vi "get_timestamp_from_distance_old.vi"(6 "distance":dbl, 9 "manual end":timestamp, 10 "start":timestamp, 11 "lat/lon position":T1) -> (1 "distance":dbl, 2 "mean speed":dbl, 3 "end times":timestamp[](array[timestamp]), 4 "time between timestamps":dbl)   [LabVIEW 2020]
uses:
  <vilib>/Analysis/1siggen.llb/Ramp Pattern by Delta.vi
  <vilib>/Analysis/NI_AALBase.lvlib
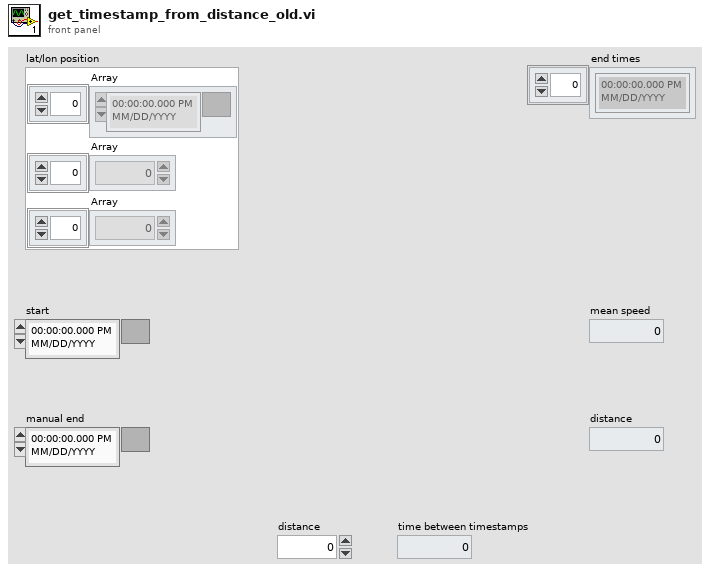
[diagram p1: front panel]
types:
  T1 = cluster{"Array":timestamp[], "Array":dbl[], "Array":dbl[]}
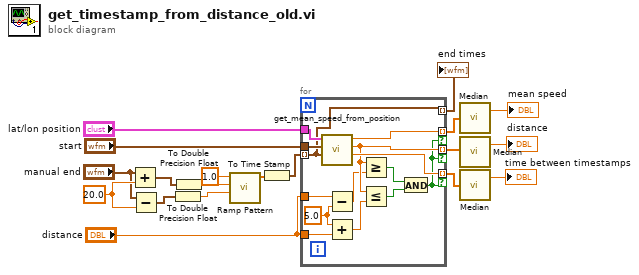
[diagram p0: block diagram]
diagram:
  w5 = 20.0 ("delta")
  n1 = Add(x="manual end", y=w5) -> (x+y=w7:timestamp)
  n2 = Subtract(x="manual end", y=w5) -> (x-y=w8:timestamp)
  n3 = To Double Precision Float(number=w8) -> (double precision float=w9:dbl)
  n4 = To Double Precision Float(number=w7) -> (double precision float=w6:dbl)
  n5 = call-poly <vilib>:"Ramp Pattern.vi"("start"=w9, "end"=w6, "delta"=1.0) -> ("Ramp Pattern"=w10:dbl[])  [unwired: 6 in, 2 out]
  n6 = To Time Stamp(1:w10) -> (0:w11:timestamp[])
  n7 = for {
    tunnel: "start" -> [w33]
    tunnel: "lat/lon position" -> [w32]
    tunnel: w11 -> [w26] mode=indexing
    tunnel: [w31] -> w13 mode=indexing if=w25
    tunnel: [w28] -> w14 mode=indexing if=w25
    tunnel: [w30] -> w15 mode=indexing if=w25
    tunnel: [w26] -> w12 mode=indexing
    tunnel: "distance" -> [w21]
    tunnel: "distance" -> [w20]
    w22 = 5.0 ("y")
    n8 = call "get_mean_speed_from_position.vi"("end"=w26, "start"=w33, "lat/lon position"=w32) -> ("dt [s]"=w30:dbl, "distance [m]"=w28:dbl, "mean speed [m/s]"=w31:dbl)  [unwired: 6 in]
    n9 = Subtract(x=w21, y=w22) -> (x-y=w23:dbl)
    n10 = Add(x=w22, y=w20) -> (x+y=w24:dbl)
    n11 = Greater Or Equal?(x=w28, y=w23) -> (x >= y?=w29:bool)
    n12 = Less Or Equal?(x=w28, y=w24) -> (x <= y?=w27:bool)
    n13 = And(x=w29, y=w27) -> (x .and. y?=w25:bool)
  }
  "end times" <- w12
  n14 = call <vilib>:"Median.vi"("X"=w13) -> ("median"=→"mean speed":dbl)  [unwired: 1 out]
  n15 = call <vilib>:"Median.vi"("X"=w14) -> ("median"=→"distance":dbl)  [unwired: 1 out]
  n16 = call <vilib>:"Median.vi"("X"=w15) -> ("median"=→"time between timestamps":dbl)  [unwired: 1 out]
